vi "DigitalINBuffserSizeSet.vi"(8 "error in (no error)":errorcluster caption="错误输入（无错误）", 10 "BufferSize":i32=2048, 11 "handle":u64) -> (0 "error out":errorcluster caption="错误输出", 2 "function return":i32, 3 "handle out":u64)   [LabVIEW 2018]
doc: "Set pos. or neg. Supply voltage"
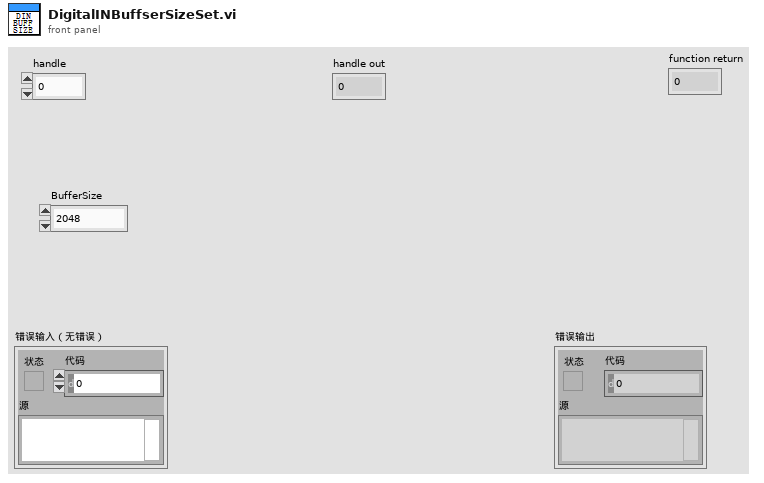
[diagram p1: front panel]
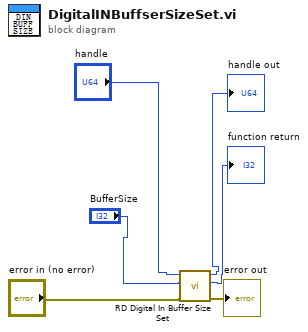
[diagram p0: block diagram]
diagram:
  n1 = call "RD Digital In Buffer Size Set.vi"("error in (no error)"="error in (no error)", "buffersize"="BufferSize", "handle"="handle") -> ("error out"=→"error out":errorcluster, "function return"=→"function return":i32, "handle out"=→"handle out":u64)  [unwired: 6 in]
